vi "instr_readModbus.vi"(8 "error in (no error)":errorcluster, 11 "Instrument in":refnum<class "Instrument.lvclass">) -> (0 "error out":errorcluster, 2 "Cluster":T1, 3 "Instrument out":refnum<class "Instrument.lvclass">)   [LabVIEW 2019, in "Instrument.lvclass"]
uses:
  Instrument.lvclass
  instr_dataCluster.ctl
  Instrument.lvclass/Instrument.ctl
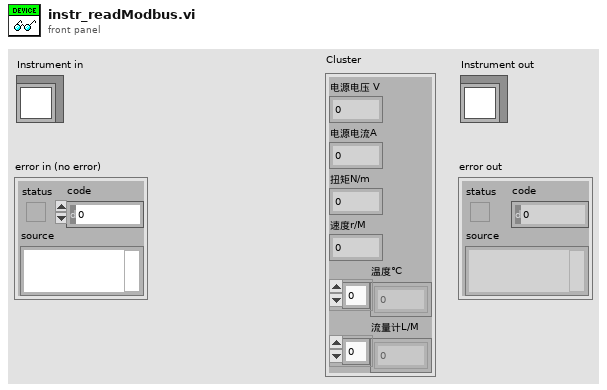
[diagram p1: front panel]
types:
  T1 = typedef "Instrument.lvclass/instr_dataCluster.ctl" = cluster{"电源电压 V":dbl, "电源电流A":dbl, "扭矩N/m":dbl, "速度r/M":dbl, "温度℃":dbl[], "流量计L/M":dbl[]}
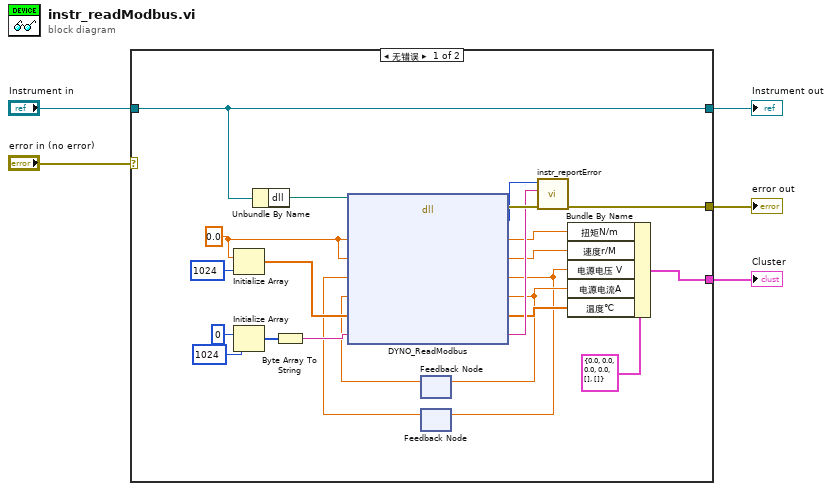
[diagram p0: block diagram]
diagram:
  n1 = case shown="无错误" "error in (no error)" {
    selector: "error in (no error)" -> [_ w29]
    tunnel: [w24 w29] -> w4
    tunnel: [w27 w28] -> w2
    tunnel: "Instrument in" -> [w27 w28]
    tunnel: [w11 _] -> w1
    frame No Error {
      w6 = 0.0 ("element")
      n2 = Initialize Array(w6, 1024 ("dimension size")) -> (w16:dbl[])
      n3 = Initialize Array(u8 0 ("element"), 1024 ("dimension size")) -> (w19:u8[])
      n4 = Unbundle By Name(w27) -> ("dll"=w26:path)
      n5 = Byte Array To String(unsigned byte array=w19) -> (string=w18:string)
      n6 = feedback #1() -> (w9:dbl)  [unwired: 1 in]
      n7 = feedback #2() -> (w7:dbl)  [unwired: 1 in]
      n8 = dll-call lib="C:/Dev/dyno/software/data/DynoAPI.dll" fn="DYNO_ReadModbus"(path in=w26, "torque"=w6, "speed"=w6, "voltage"=w7, "current"=w9, "temperature"=w16, "errorMsg"=w18) -> (error out=w25:errorcluster, "return type"=w23:i32, "torque"=w14:dbl, "speed"=w13:dbl, "voltage"=w8:dbl, "current"=w10:dbl, "temperature"=w12:dbl[], "errorMsg"=w22:string)  [unwired: 2 in, 1 out]
      n9 = feedback-in #1(w10) -> ()
      n10 = feedback-in #2(w8) -> ()
      n11 = call "instr_reportError.vi"("error in (no error)"=w25, "errorMsg"=w22, "return type"=w23) -> ("error out"=w24:errorcluster)  [unwired: 8 in]
      n12 = Bundle By Name(cluster=T1 {"电源电压 V"=0.0, "电源电流A"=0.0, "扭矩N/m"=0.0, "速度r/M"=0.0, "温度℃"=[], "流量计L/M"=[]} ("Cluster"), "扭矩N/m"=w14, "速度r/M"=w13, "电源电压 V"=w8, "电源电流A"=w10, "温度℃"=w12) -> (w11:T1)
    }
    frame Error {
    }
  }
  "error out" <- w4
  "Instrument out" <- w2
  "Cluster" <- w1
